vi "Delete Directory.vi"(8 "error in (no error)":errorcluster, 10 "Remote Directory":string, 11 "FTP in":refnum<class "FTP.lvclass">) -> (0 "error out":errorcluster, 3 "FTP out":refnum<class "FTP.lvclass">)   [LabVIEW 2017, in "FTP.lvlib" / "FTP.lvclass"]
uses:
  FTP.lvclass
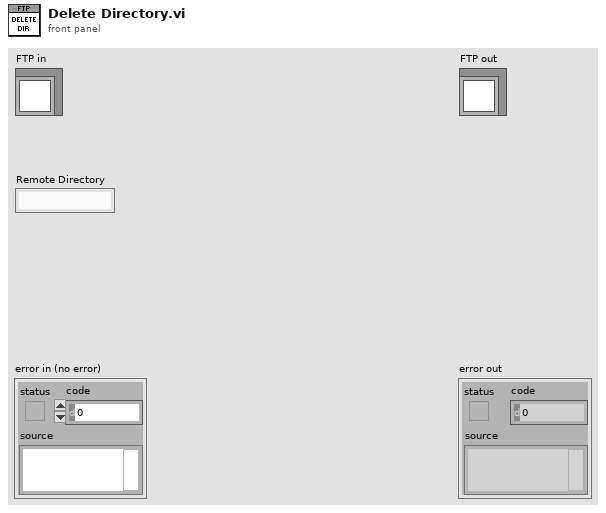
[diagram p1: front panel]
types:
  T1 = typedef "FTP.lvlib/FTP.lvclass/Dir-File Info.ctl" = cluster{"Name":string, "Modify Timestamp":timestamp, "Dir-File Type":T2, "Unique Id":string, "Permissions":string, "Unix Mode":u16, "Owner":string, "Group":string, "FileSize":i64}
  T2 = typedef "FTP.lvlib/FTP.lvclass/Dir-File Type.ctl" = enum16{"File", "Listed Directory", "Parent Directory", "Directory", "Unknown"}
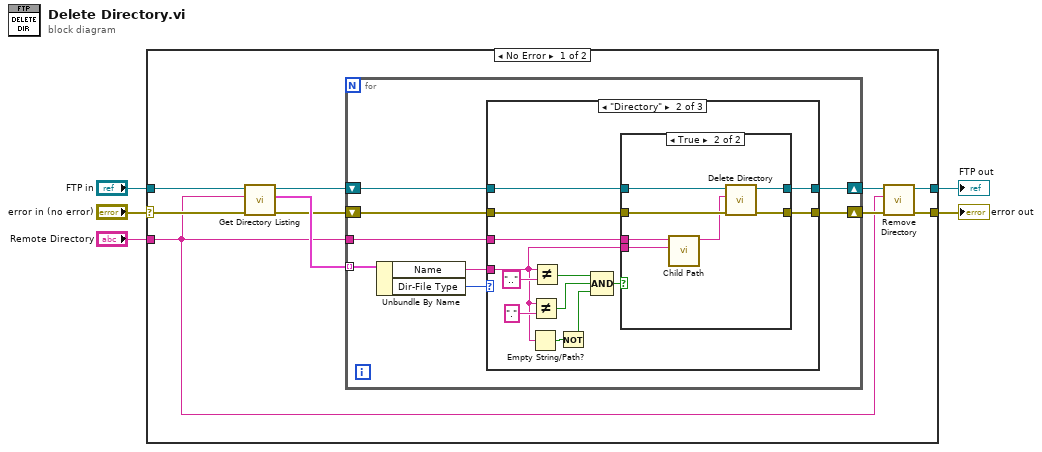
[diagram p0: block diagram]
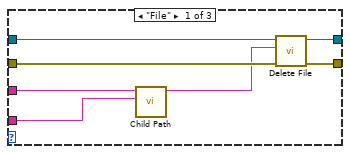
[diagram p2: hidden frame]
diagram:
  n1 = case shown="No Error" "error in (no error)" {
    selector: "error in (no error)" -> [w14 w56]
    tunnel: [w7 w56] -> w4
    tunnel: [w8 w55] -> w2
    tunnel: "FTP in" -> [w15 w55]
    tunnel: "Remote Directory" -> [w6 _]
    frame No Error {
      n2 = call "Get Directory Listing.vi"("error in (no error)"=w14, "RemoteDirectory"=w6, "FTP in"=w15) -> ("error out"=w11:errorcluster, "Dir-File Info Array"=w12:T1[], "FTP out"=w13:refnum<class "FTP.lvclass">)  [unwired: 6 in]
      n3 = for {
        shift-right: [w18] -> w10
        shift-left: w13 -> [w21]
        tunnel: w12 -> [w23] mode=indexing
        tunnel: w6 -> [w19]
        shift-right: [w16] -> w9
        shift-left: w11 -> [w17]
        n4 = Unbundle By Name(w23) -> ("Name"=w20:string, "Dir-File Type"=w22:T2)
        n5 = case shown="\"Directory\"" w22 {
          tunnel: w21 -> [w30 w37 w54]
          tunnel: w20 -> [w25 w32 _]
          tunnel: w19 -> [w26 w33 _]
          tunnel: [w29 w36 w54] -> w18
          tunnel: w17 -> [w28 w35 w53]
          tunnel: [w27 w34 w53] -> w16
          frame "File" {
            n6 = call "Child Path.vi"("Name"=w25, "Remote Directory"=w26) -> ("String"=w24:string)  [unwired: 9 in]
            n7 = call "Delete File.vi"("error in (no error)"=w28, "RemoteFileName"=w24, "FTP in"=w30) -> ("error out"=w27:errorcluster, "FTP out"=w29:refnum<class "FTP.lvclass">)  [unwired: 7 in]
          }
          frame "Directory" {
            n8 = Empty String/Path?(string/path=w32) -> (empty?=w39:bool)
            n9 = Not Equal?(x=w32, y=".") -> (x != y?=w40:bool)
            n10 = Not Equal?(x=w32, y="..") -> (x != y?=w41:bool)
            n11 = Not(x=w39) -> (.not. x?=w31:bool)
            n12 = Compound Arithmetic op=AND(w41, w40, w31) -> (w38:bool)
            n13 = case shown="True" w38 {
              tunnel: w37 -> [w45 w52]
              tunnel: [w45 w51] -> w36
              tunnel: w35 -> [w44 w50]
              tunnel: [w44 w49] -> w34
              tunnel: w33 -> [_ w48]
              tunnel: w32 -> [_ w47]
              frame False {
              }
              frame True {
                n14 = call "Child Path.vi"("Name"=w47, "Remote Directory"=w48) -> ("String"=w46:string)  [unwired: 9 in]
                n15 = call "Delete Directory.vi"("error in (no error)"=w50, "Remote Directory"=w46, "FTP in"=w52) -> ("error out"=w49:errorcluster, "FTP out"=w51:refnum<class "FTP.lvclass">)  [unwired: 7 in]
              }
            }
          }
          frame Default {
          }
        }
      }
      n16 = call "Remove Directory.vi"("error in (no error)"=w9, "Remote Directory"=w6, "FTP in"=w10) -> ("error out"=w7:errorcluster, "FTP out"=w8:refnum<class "FTP.lvclass">)  [unwired: 7 in]
    }
    frame Error {
    }
  }
  "error out" <- w4
  "FTP out" <- w2
